vi "Engine-DI-CalTablesB.vi"(4 "RailP [bar]":sgl, 6 "InjQty [mm3/stroke]":sgl, 8 "Injector":i32, 11 "Aux IDs":fxp<+,4,4>) -> (3 "Durations [s]":sgl)   [LabVIEW 2016, in "DSI-RT.lvlib"]
uses:
  DSI-RT.lvlib
  <vilib>/addons/Software Calibration Management/xSCM/Controls/TLU2D.ctl
  <vilib>/addons/Software Calibration Management/xSCM/Controls/TBL2D.ctl
  <vilib>/addons/Software Calibration Management/xSCM/CalPoint.xnode
  <vilib>/addons/Software Calibration Management/xSCM/SCM-API.lvlib
  <vilib>/addons/Software Calibration Management/xSCM/ni_scm.dll
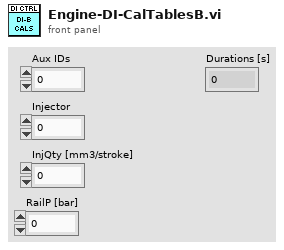
[diagram p1: front panel]
types:
  T1 = typedef "SCM-API.lvlib/TBL2D.ctl" = cluster{"X":sgl[], "Y":sgl[], "Z":sgl[][]}
  T2 = typedef "SCM-API.lvlib/TLU2D.ctl" = cluster{"X":sgl, "Y":sgl, "Z":sgl}
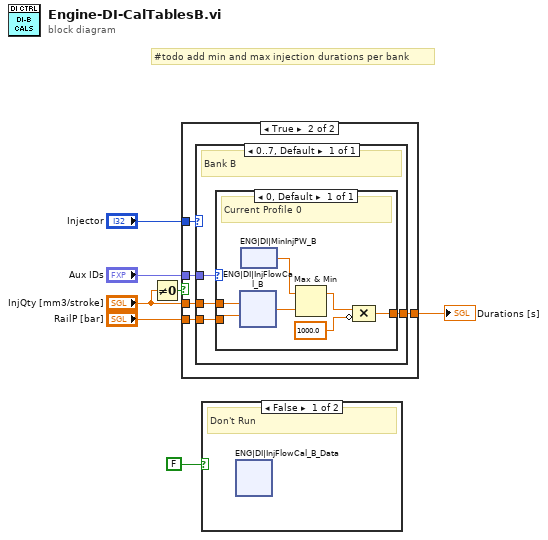
[diagram p0: block diagram]
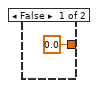
[diagram p3: hidden frame]
diagram:
  # "#todo add min and max injection durations per bank"
  n1 = Not Equal To 0?(x="InjQty [mm3/stroke]") -> (x != 0?=w1:bool)
  n2 = case shown="True" w1 {
    tunnel: "Injector" -> [_ w13]
    tunnel: "Aux IDs" -> [_ w12]
    tunnel: [sgl 0.0 ("Z") w11] -> w5
    tunnel: "RailP [bar]" -> [_ w10]
    tunnel: "InjQty [mm3/stroke]" -> [_ w9]
    frame False {
    }
    frame True {
      n3 = case shown="0..7, Default" w13 {
        tunnel: w12 -> [w17]
        tunnel: [w16] -> w11
        tunnel: w10 -> [w15]
        tunnel: w9 -> [w14]
        frame 0..7, Default {
          # "Bank B"
          n4 = case shown="0, Default" w17 {
            tunnel: [w21] -> w16
            tunnel: w15 -> [w23]
            tunnel: w14 -> [w22]
            frame 0, Default {
              # "Current Profile 0"
              n5 = xnode "ENG|DI|InjFlowCal_B"("Y Index"=w23, "X Index"=w22) -> ("Z"=w24:sgl)
              n6 = xnode "ENG|DI|MinInjPW_B"() -> ("Value"=w18:sgl)
              n7 = Max & Min(x=w18, y=w24) -> (max(x,y)=w19:sgl)  [unwired: 1 out]
              n8 = Compound Arithmetic op=MULTIPLY(w19, invert sgl 1000.0 ("value")) -> (w21:sgl)
            }
          }
        }
      }
    }
  }
  "Durations [s]" <- w5
  n9 = case shown="False" FALSE {
    frame False {
      # "Don't Run"
      n10 = xnode "ENG|DI|InjFlowCal_B_Data"() -> ()  [unwired: 1 out]
    }
    frame True {
    }
  }
